vi "Add_TTL_IO_times-to-live.vi"(8 "error in (no error)":errorcluster, 9 "Data to update":T1[](array[typedef]), 10 "IO ports status in":T2, 11 "Previous loop time, us":i32) -> (0 "error out":errorcluster, 3 "IO ports status out":i32[][](array[numeric]))   [LabVIEW 2018, in "TTL IO.lvlib"]
uses:
  TTL IO.lvlib
  Typedefs/CTL_IO_ports_status.ctl
  Typedefs/CTL_TTL_command_block.ctl
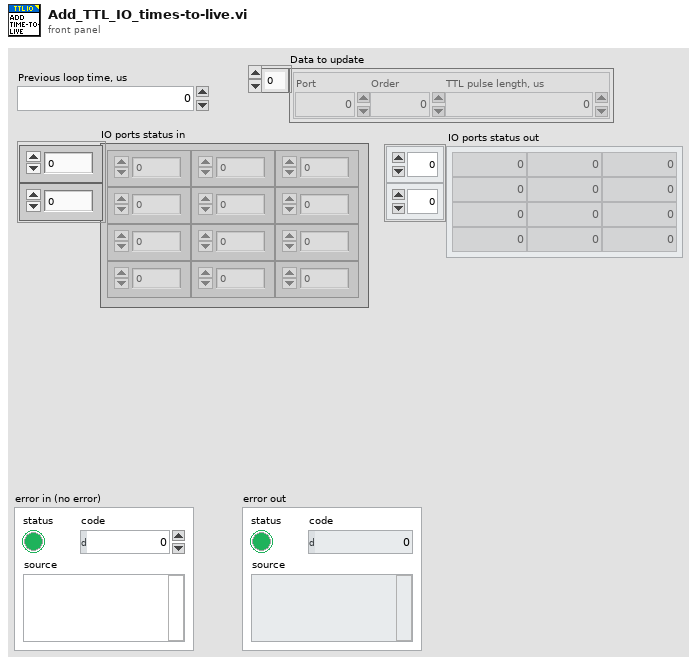
[diagram p1: front panel]
types:
  T1 = typedef "TTL IO.lvlib/CTL_TTL_command_block.ctl" = cluster{"Port":i16, "Order":i32, "TTL pulse length, us":i32}
  T2 = typedef "TTL IO.lvlib/CTL_IO_ports_status.ctl" = i32[][]
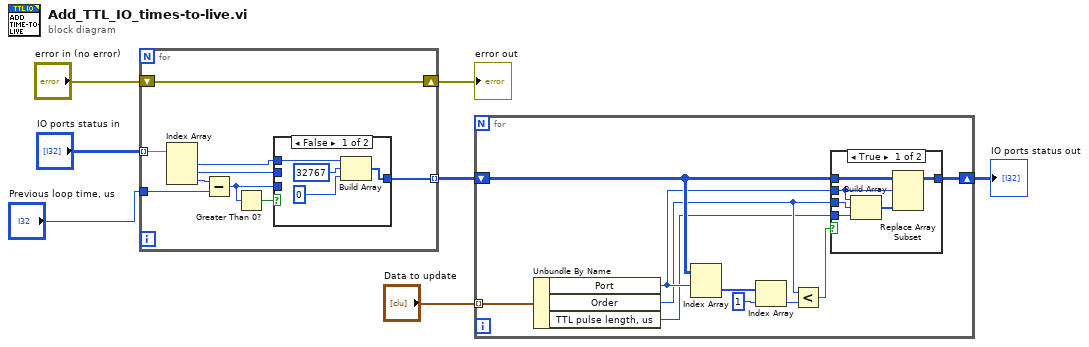
[diagram p0: block diagram]
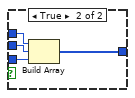
[diagram p3: hidden frame]
diagram:
  n1 = for {
    tunnel: "Previous loop time, us" -> [w14]
    shift-right: [w8] -> w7
    shift-left: "error in (no error)" -> [w8]
    tunnel: "IO ports status in" -> [w16] mode=indexing
    tunnel: [w9] -> w2 mode=indexing
    n2 = Index Array(array=w16) -> (element #1=w10:i32, element #2=w11:i32, element #3=w15:i32)  [unwired: 3 in]
    n3 = Subtract(x=w15, y=w14) -> (x-y=w12:i32)
    n4 = Greater Than 0?(x=w12) -> (x > 0?=w13:bool)
    n5 = case shown="False" w13 {
      tunnel: w12 -> [_ w22]
      tunnel: w11 -> [_ w23]
      tunnel: w10 -> [w20 w24]
      tunnel: [w17 w21] -> w9
      frame False {
        n6 = Build Array(w20, 32767 ("element"), 0 ("element")) -> (w17:i32[])
      }
      frame True {
        n7 = Build Array(w24, w23, w22) -> (w21:i32[])
      }
    }
  }
  "error out" <- w7
  n8 = for {
    tunnel: "Data to update" -> [w34] mode=indexing
    shift-right: [w30] -> w1
    shift-left: w2 -> [w31]
    n9 = Unbundle By Name(w34) -> ("Port"=w29:i16, "Order"=w28:i32, "TTL pulse length, us"=w27:i32)
    n10 = Index Array(array=w31, index (row)=w29) -> (element=w33:i32[])  [unwired: 1 in]
    n11 = Index Array(array=w33, index=1) -> (element=w25:i32)
    n12 = Less?(x=w28, y=w25) -> (x < y?=w32:bool)
    n13 = case shown="True" w32 {
      tunnel: w31 -> [w40 w41]
      tunnel: [w39 w41] -> w30
      tunnel: w29 -> [w38 _]
      tunnel: w28 -> [w37 _]
      tunnel: w27 -> [w36 _]
      frame True {
        n14 = Build Array(w38, w37, w36) -> (w35:i32[])
        n15 = Replace Array Subset(array=w40, new element=w35, index (row)=w38) -> (w39:i32[][])  [unwired: 1 in]
      }
      frame False {
      }
    }
  }
  "IO ports status out" <- w1
